vi "FGV Stickstoff Befuellung.vi"(8 "Aktion":T2=enum."Befüllen vorbereiten", 11 "Stiskstoff Befüllzeiten":T1) -> (0 "Ausgang":bool, 1 "Befülldauer":sgl, 2 "Befüllen 2":timestamp, 3 "Befüllen 1":timestamp, 4 "Warten/Befüllzeit":dbl, 5 "Timeout":bool, 6 "Aktion":T2=enum."Befüllen vorbereiten")   [LabVIEW 2020, in "Stickstoff Befuellung.lvlib"]
uses:
  Stickstoff Befuellung.lvlib
  Aktionen Stockstoff Befuellung.ctl
  Stickstoff Befuellzeiten.ctl
  Konfig-Dateien/FGV Betriebsdaten Aktionen.ctl
  Verwaltung/FGV IN Aktionen.ctl
  Allgemein/Allgemein.lvlib
  Konfig-Dateien/Konfig-Dateien.lvlib
  Verwaltung/Verwaltung - cRIO.lvlib
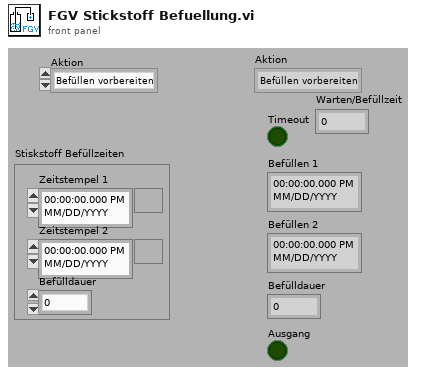
[diagram p1: front panel]
types:
  T1 = typedef "Stickstoff Befuellung.lvlib/Stickstoff Befuellzeiten.ctl" = cluster{"Zeitstempel 1":timestamp, "Zeitstempel 2":timestamp, "Befülldauer":sgl}
  T2 = typedef "Stickstoff Befuellung.lvlib/Aktionen Stockstoff Befuellung.ctl" = enum16{"lesen", "Befüllen vorbereiten", "Befüllen", "Befüllen beenden", "Warten", "deaktiviert", "initialisieren", "anstehender Fehler"}
  T3 = typedef "Verwaltung - cRIO.lvlib/FGV IN Aktionen.ctl" = enum16{"lesen", "DI", "AI", "Fühler Br.", "TC", "Fühler Br. TC"}
  T4 = typedef "Konfig-Dateien.lvlib/FGV Betriebsdaten Aktionen.ctl" = enum16{"lesen", "Anlagengrenzw.", "PID Param.", "Sonstige", "Sensor Para."}
  T5 = typedef "Verwaltung - cRIO.lvlib/Digital Eingaenge 0-15.ctl" = cluster{"I0: N2 Nachf. FT-IR voll":bool, "I1: N2 Nachf. Vorrat leer":bool, "I2: (Klimaanlage eingeschaltet)":bool, "I3: (Klimaanlage Störung)":bool, "I4: Trigger Eingang (Messdaten sp.)":bool, "I5: Reserve":bool, "I6: Reserve":bool, "I7: Reserve":bool, "I8: Druckschalter Versorgung ok":bool, "I9: Reserve":bool, "I10: Reserve":bool, "I11: Reserve":bool, "I12: Drucksch. N2 Versorgung":bool, "I13: Reserve":bool, "I14: Drucksch. N2 Optikbox":bool, "I15: (Füllstand Kondensatbehälter)":bool}
  T6 = typedef "Erweiterte Konfig.lvlib/Sonstige Parameter.ctl" = cluster{"Lüfter langsam":sgl, "Lüfter schnell":sgl, "FT-IR Kühlung Soll":sgl, "FT-IR Kühlung Max":sgl, "Überwachung":T7, "Befüllung aktiv":T8, "Stickstoff Befüllzeit":sgl, "Befüllintervall":sgl, "Kalibrierwert FT-IR":sgl, "Offset Ausgang":sgl, "Offset FT-IR":sgl, "Offset Druck FT-IR":sgl, "Dichtheitstest Zeit":sgl, "Dichtheitstest Abfall":sgl, "Dichtheitstest Umfang":T9, "Offset Umgebung":sgl, "Max Taupunkt":sgl, "Pumpendrehzahl":sgl, "ext. Befüllung":T8, "Ext. Stickstoff Befüllzeit":sgl}
  T7 = typedef "Auswahlfeld.ctl" = u16
  T8 = typedef "LogKonfig.lvlib/Auswahlfeld aktiviert-deaktiviert.ctl" = u16
  T9 = typedef "Erweiterte Konfig.lvlib/Dichtheitstest Umfang.ctl" = u16
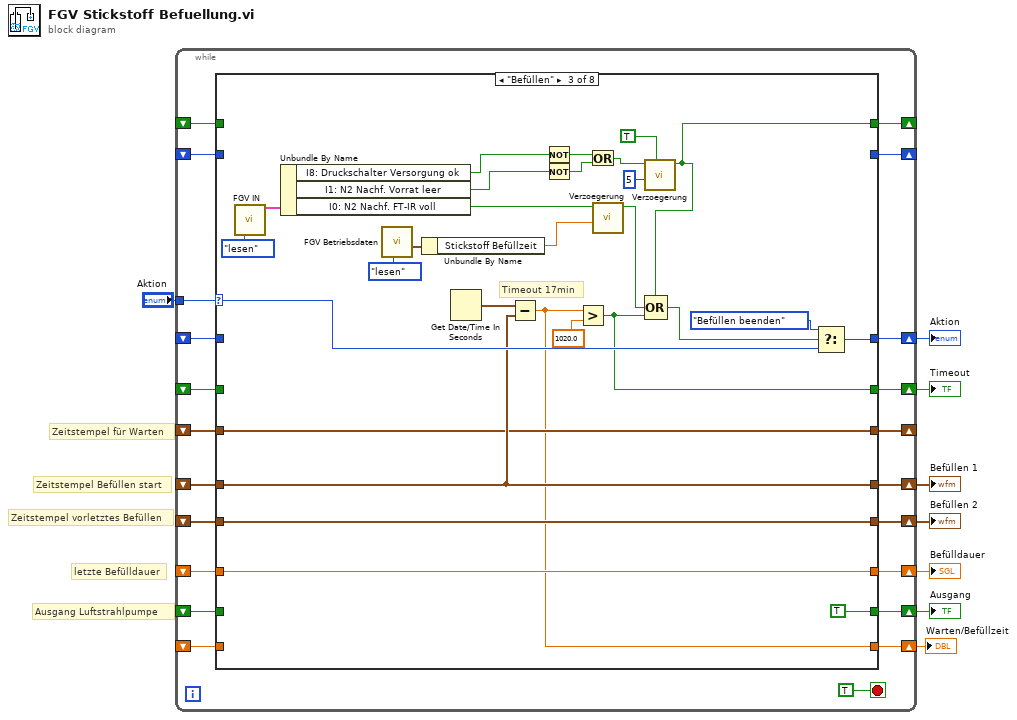
[diagram p0: block diagram]
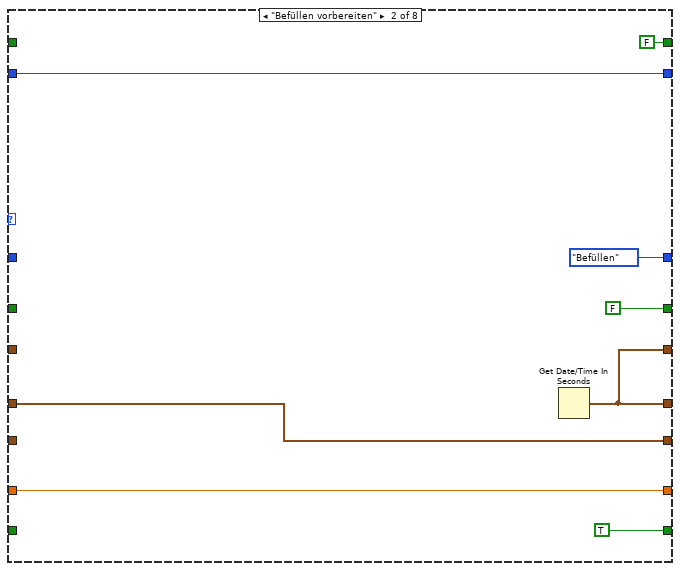
[diagram p3: hidden frame]
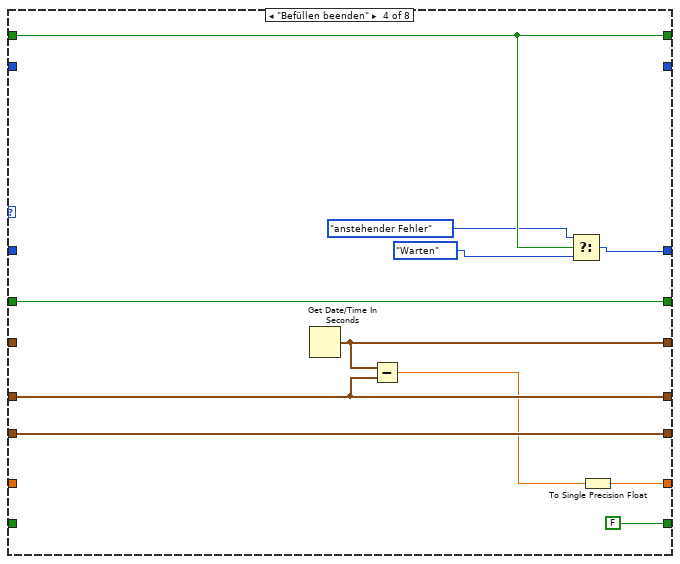
[diagram p4: hidden frame]
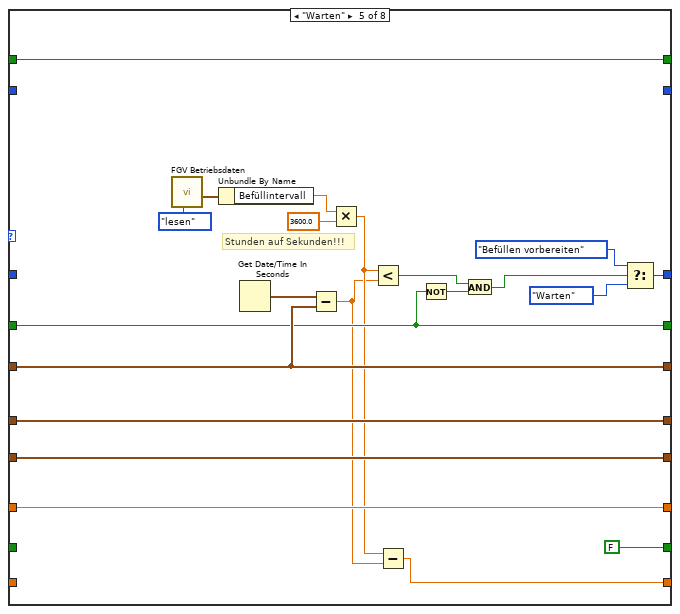
[diagram p5: hidden frame]
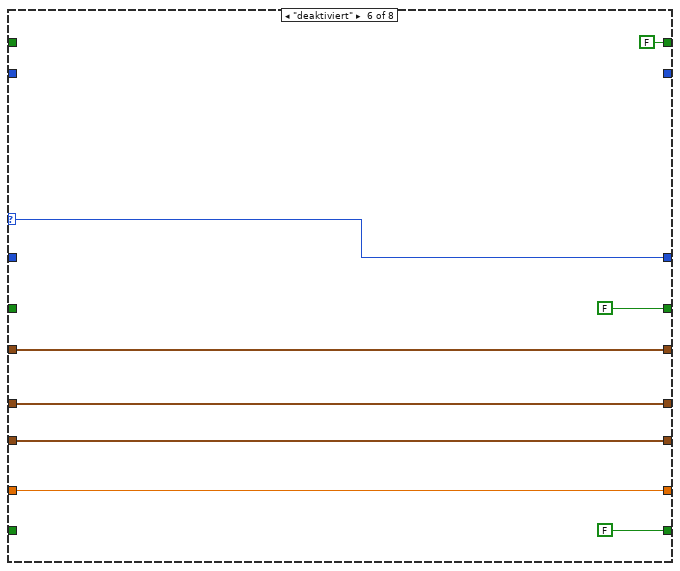
[diagram p6: hidden frame]
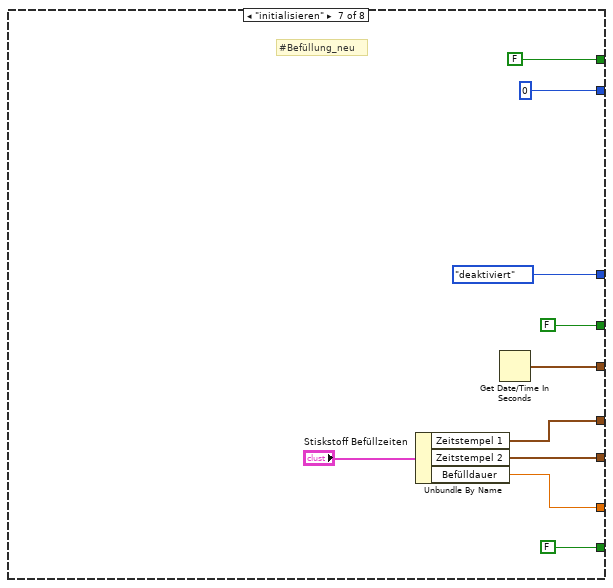
[diagram p7: hidden frame]
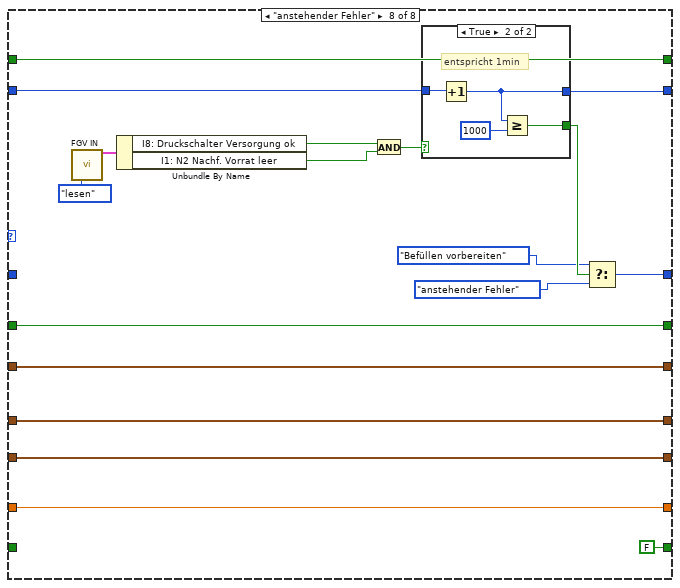
[diagram p8: hidden frame]
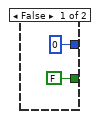
[diagram p9: hidden frame]
diagram:
  # "Zeitstempel für Warten"
  # "Ausgang Luftstrahlpumpe"
  # "Zeitstempel vorletztes Befüllen"
  # "letzte Befülldauer"
  # "Zeitstempel Befüllen start"
  n1 = while {
    tunnel: "Aktion" -> [w27]
    shift-right: [w24] -> w7
    shift-left: _ -> [w22]
    shift-right: [w28] -> w5
    shift-left: _ -> [w20]
    shift-right: [w23] -> w6
    shift-left: _ -> [w21]
    shift-right: [w29] -> w4
    shift-left: _ -> [w19]
    shift-right: [w25] -> w8
    shift-left: _ -> [w18]
    shift-right: [w26] -> w3
    shift-left: _ -> [w17]
    shift-right: [w15] -> _
    shift-left: _ -> [w16]
    shift-right: [w14] -> _
    shift-left: _ -> [w13]
    shift-right: [w12] -> _
    shift-left: _ -> [w11]
    shift-right: [w10] -> w1
    shift-left: _ -> [w9]
    stop <- TRUE stop-if-true
    n2 = case shown="\"Befüllen\"" w27 {
      selector: w27 -> [_ _ w74 _ _ w116 _ _]
      tunnel: [w35 Aktionen_Stockstoff_Befuellung."Befüllen" ("Aktion") w67 w77 w101 w116 Aktionen_Stockstoff_Befuellung."deaktiviert" ("Aktion") w129] -> w26
      tunnel: [w40 w43 w70 w85 w106 w114 w124 w141] -> w24
      tunnel: [w37 TRUE TRUE FALSE FALSE FALSE FALSE FALSE] -> w29
      tunnel: w22 -> [w40 w46 w70 w85 w106 w114 _ w141]
      tunnel: [w38 w45 w71 w81 w102 w112 w125 w143] -> w28
      tunnel: w20 -> [w38 w45 w71 _ w102 w112 _ w143]
      tunnel: [w39 w46 w72 w86 w107 w113 w123 w142] -> w23
      tunnel: w21 -> [w39 _ w72 w86 w107 w113 _ w142]
      tunnel: w19 -> [w37 _ _ _ _ _ _ _]
      tunnel: [w36 FALSE w64 w84 w94 FALSE FALSE w139] -> w25
      tunnel: w18 -> [w36 _ _ w84 w94 _ _ w139]
      tunnel: w17 -> [w35 _ _ _ _ _ _ _]
      tunnel: w16 -> [w34 _ w63 _ w100 w110 _ w140]
      tunnel: [w34 w43 w63 w83 w100 w110 w119 w140] -> w15
      tunnel: [w33 FALSE ("Zeit abgelaufen?") w50 w80 w91 FALSE ("Zeit abgelaufen?") FALSE w127] -> w14
      tunnel: w13 -> [w33 _ _ w80 w91 _ _ w127]
      tunnel: [w32 w41 _ _ _ _ 0 w132] -> w12
      tunnel: w11 -> [w32 w41 _ _ _ _ _ w133]
      tunnel: [w31 _ w49 _ w88 _ _ _] -> w10
      tunnel: w9 -> [w31 _ _ _ _ _ _ _]
      frame "lesen", Default {
      }
      frame "Befüllen vorbereiten" {
        n3 = Get Date/Time In Seconds() -> (seconds since 1Jan1904=w43:timestamp)
      }
      frame "Befüllen" {
        # "Timeout 17min"
        n4 = call "FGV IN.vi"("Aktion"=FGV_IN_Aktionen."lesen") -> ("DI"=w59:T5)  [unwired: 10 in, 4 out]
        n5 = Unbundle By Name(w59) -> ("I8: Druckschalter Versorgung ok"=w51:bool, "I1: N2 Nachf. Vorrat leer"=w52:bool, "I0: N2 Nachf. FT-IR voll"=w58:bool)
        n6 = call "FGV Betriebsdaten.vi"("Aktionen"=FGV_Betriebsdaten_Aktionen."lesen") -> ("Sonstige"=w61:T6)  [unwired: 7 in, 3 out]
        n7 = Unbundle By Name(w61) -> ("Stickstoff Befüllzeit"=w76:sgl)
        n8 = Get Date/Time In Seconds() -> (seconds since 1Jan1904=w69:timestamp)
        n9 = Subtract(x=w69, y=w70) -> (x-y=w49:dbl)
        n10 = Not(x=w51) -> (.not. x?=w55:bool)
        n11 = Not(x=w52) -> (.not. x?=w56:bool)
        n12 = Greater?(x=w49, y=1020.0) -> (0:w64:bool)
        n13 = Or(x=w55, y=w56) -> (x .or. y?=w57:bool)
        n14 = call "Verzoegerung.vi"("sec"=w76, "Startsignal"=w58) -> ("Zeit abgelaufen?"=w66:bool)  [unwired: 8 in, 1 out]
        n15 = call "Verzoegerung.vi"("Abfallverzögerung?"=TRUE, "sec"=u16 5, "Startsignal"=w57) -> ("Zeit abgelaufen?"=w50:bool)  [unwired: 7 in, 1 out]
        n16 = Compound Arithmetic op=OR ("Mehrfacharithmetik")(w50, w66, w64) -> (w65:bool)
        n17 = Select(t=Aktionen_Stockstoff_Befuellung."Befüllen beenden", s=w65, f=w74) -> (s? t:f=w67:T2)
      }
      frame "Befüllen beenden" {
        n18 = Get Date/Time In Seconds() -> (seconds since 1Jan1904=w83:timestamp)
        n19 = Subtract(x=w83, y=w85) -> (x-y=w82:dbl)
        n20 = Select(t=Aktionen_Stockstoff_Befuellung."anstehender Fehler" ("Aktion"), s=w80, f=Aktionen_Stockstoff_Befuellung."Warten" ("Aktion")) -> (s? t:f=w77:T2)
        n21 = To Single Precision Float(number=w82) -> (single precision float=w81:sgl)
      }
      frame "Warten" {
        # "Stunden auf Sekunden!!!"
        n22 = call "FGV Betriebsdaten.vi"("Aktionen"=FGV_Betriebsdaten_Aktionen."lesen") -> ("Sonstige"=w92:T6)  [unwired: 7 in, 3 out]
        n23 = Unbundle By Name(w92) -> ("Befüllintervall"=w99:sgl)
        n24 = Get Date/Time In Seconds() -> (seconds since 1Jan1904=w105:timestamp)
        n25 = Subtract(x=w105, y=w100) -> (x-y=w89:dbl)
        n26 = Multiply(x=w99, y=sgl 3600.0) -> (x*y=w90:sgl)
        n27 = Less?(x=w90, y=w89) -> (x < y?=w95:bool)
        n28 = Subtract(x=w90, y=w89) -> (x-y=w88:dbl)
        n29 = Not(x=w94) -> (.not. x?=w97:bool)
        n30 = And(x=w95, y=w97) -> (x .and. y?=w96:bool)
        n31 = Select(t=Aktionen_Stockstoff_Befuellung."Befüllen vorbereiten" ("Aktion"), s=w96, f=Aktionen_Stockstoff_Befuellung."Warten") -> (s? t:f=w101:T2)
      }
      frame "deaktiviert" {
      }
      frame "initialisieren" {
        # "#Befüllung_neu"
        n32 = Unbundle By Name("Stiskstoff Befüllzeiten") -> ("Zeitstempel 1"=w124:timestamp, "Zeitstempel 2"=w123:timestamp, "Befülldauer"=w125:sgl)
        n33 = Get Date/Time In Seconds() -> (seconds since 1Jan1904=w119:timestamp)
      }
      frame "anstehender Fehler" {
        n34 = call "FGV IN.vi"("Aktion"=FGV_IN_Aktionen."lesen") -> ("DI"=w137:T5)  [unwired: 10 in, 4 out]
        n35 = Unbundle By Name(w137) -> ("I8: Druckschalter Versorgung ok"=w136:bool, "I1: N2 Nachf. Vorrat leer"=w135:bool)
        n36 = And(x=w136, y=w135) -> (x .and. y?=w134:bool)
        n37 = case shown="True" w134 {
          tunnel: w133 -> [_ w150]
          tunnel: [0 w149] -> w132
          tunnel: [FALSE w147] -> w131
          frame False {
          }
          frame True {
            # "entspricht 1min"
            n38 = Increment(x=w150) -> (x+1=w149:i32)
            n39 = Greater Or Equal?(x=w149, y=1000) -> (x >= y?=w147:bool)
          }
        }
        n40 = Select(t=Aktionen_Stockstoff_Befuellung."Befüllen vorbereiten", s=w131, f=Aktionen_Stockstoff_Befuellung."anstehender Fehler" ("Aktion")) -> (s? t:f=w129:T2)
      }
    }
  }
  "Aktion" <- w3
  "Timeout" <- w8
  "Befüllen 1" <- w7
  "Befüllen 2" <- w6
  "Befülldauer" <- w5
  "Ausgang" <- w4
  "Warten/Befüllzeit" <- w1
